vi "DB Close.vi"(8 "error in":errorcluster, 11 "Database in":refnum<class "MYSQL Database.lvclass">) -> (0 "error out":errorcluster, 3 "Database out":refnum<class "MYSQL Database.lvclass">)   [LabVIEW 2023, in "HardwareAbstractionLayer_LVOOP.lvlib" / "MYSQL Database.lvclass"]
doc: "This VI is Database Close Reference"
uses:
  MYSQL Database.lvclass
  MYSQL Database.lvclass/MYSQL Database.ctl
  <vilib>/addons/database/NI_Database_API.lvlib
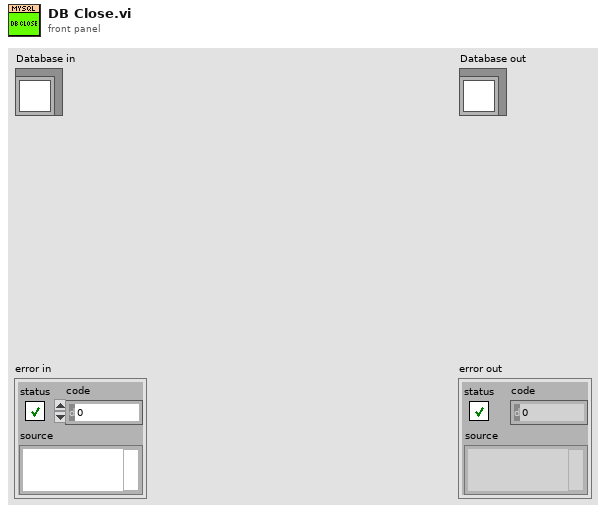
[diagram p1: front panel]
types:
  T1 = typedef "NI_Database_API.lvlib/Conn ObjectReference.ctl" = refnum<k1>
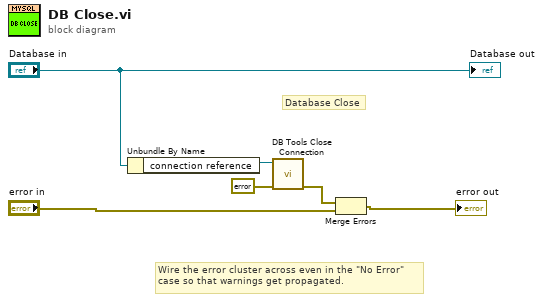
[diagram p0: block diagram]
diagram:
  # "Database Close"
  # "Wire the error cluster across even in the \"No Error\"\ncase so that warnings get propagated."
  n1 = Unbundle By Name("Database in") -> ("connection reference"=w3:T1)
  n2 = call <vilib>:"DB Tools Close Connection.vi"("error in (no error)"=errorcluster {"status"=FALSE, "code"=0, "source"=""}, "connection reference"=w3) -> ("error out"=w2:errorcluster)  [unwired: 5 in]
  n3 = Merge Errors(w2, "error in") -> (→"error out":errorcluster)
  "Database out" <- "Database in"
